vi "adpm ap set max latency value seconds.vi"(10 "max_latency_seconds":u16, 11 "ap_handle":u32) -> (2 "function return":i32, 3 "ap_handle out":u32)   [LabVIEW 2019, in "apdm.lvlib"]
doc: "APDM_EXPORT int adpm_ap_set_max_latency_value_seconds(apdm_ap_handle_t ap_handle, const uint16_t max_latency_seconds);"
uses:
  apdm.lvlib
  Lee Lab/CP FES Walking 2018/Code/Working/LabVIEW/apdm.dll
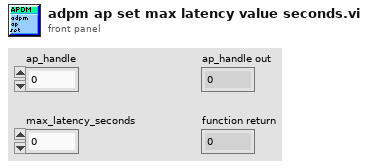
[diagram p1: front panel]
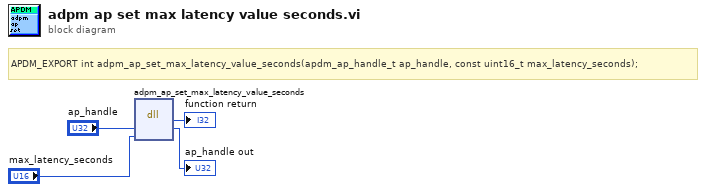
[diagram p0: block diagram]
diagram:
  # "APDM_EXPORT int adpm_ap_set_max_latency_value_seconds(apdm_ap_handle_t ap_handle, const uint16_t max_latency_seconds);"
  n1 = dll-call lib="C:/Users/jfalesi/Dropbox/Lee Lab/CP FES Walking 2018/Code/Working/LabVIEW/apdm.*" fn="adpm_ap_set_max_latency_value_seconds"("ap_handle"="ap_handle", "max_latency_seconds"="max_latency_seconds") -> (→"function return":i32, "ap_handle"=→"ap_handle out":u32)  [unwired: 4 in, 2 out]
